vi "Log File.vi"(8 "Error In":errorcluster, 10 "Model (F-ME74)":bool, 11 "Test Data table":refnum<vi>) -> (0 "Error Out":errorcluster)   [LabVIEW 2018]
uses:
  <vilib>/Utility/file.llb/Write Delimited Spreadsheet (string).vi
panel:
  # "LOG File"
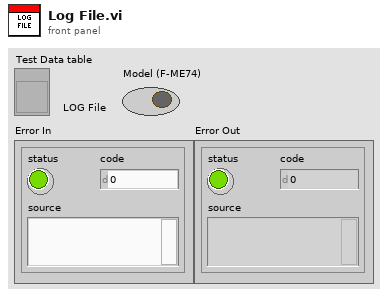
[diagram p1: front panel]
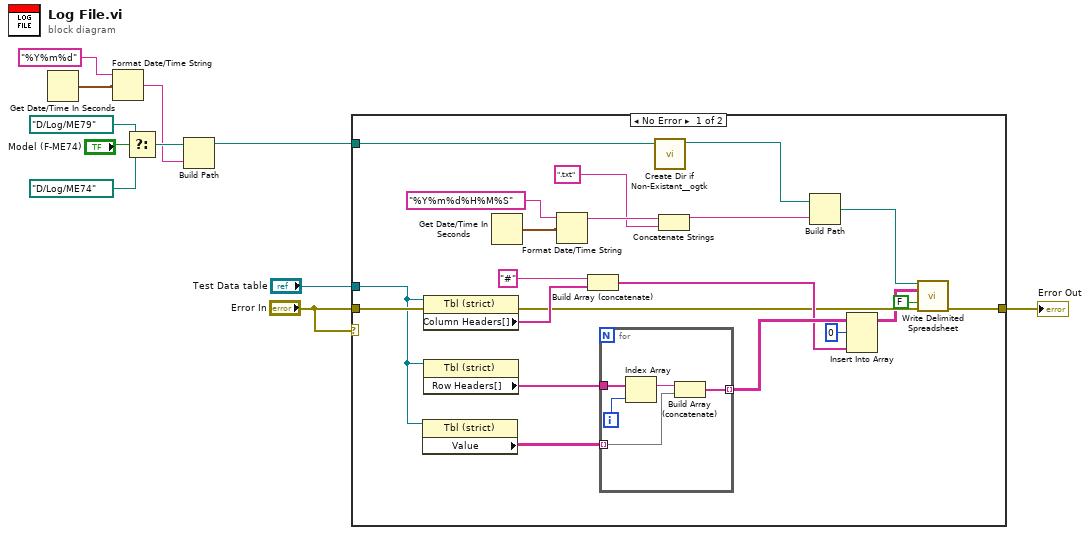
[diagram p0: block diagram]
diagram:
  n1 = Get Date/Time In Seconds() -> (seconds since 1Jan1904=w4:timestamp)
  n2 = Format Date/Time String(time format string (%c)="%Y%m%d", seconds (now)=w4) -> (date/time string=w2:string)  [unwired: 1 in]
  n3 = Select(t=path "D:/Log/ME79" ("base path"), s="Model (F-ME74)", f=path "D:/Log/ME74" ("base path")) -> (s? t:f=w3:path)
  n4 = Build Path(base path=w3, name or relative path=w2) -> (appended path=w1:path)
  n5 = case shown="No Error" "Error In" {
    tunnel: "Error In" -> [w32 w38]
    tunnel: "Test Data table" -> [w22 _]
    tunnel: [w21 w38] -> w10
    tunnel: w1 -> [w14 _]
    frame No Error {
      n6 = property class="Tbl (strict)"(reference=w22) -> ("Value"=w28:string[][])  [unwired: 1 in, 2 out]
      n7 = property class="Tbl (strict)"(reference=w22, error in=w32) -> (error out=w24:errorcluster, "Column Headers[]"=w30:string[])  [unwired: 1 out]
      n8 = property class="Tbl (strict)"(reference=w22) -> ("Row Headers[]"=w29:string[])  [unwired: 1 in, 2 out]
      n9 = Get Date/Time In Seconds() -> (seconds since 1Jan1904=w20:timestamp)
      n10 = Format Date/Time String(time format string (%c)="%Y%m%d%H%M%S", seconds (now)=w20) -> (date/time string=w18:string)  [unwired: 1 in]
      n11 = Build Array (concatenate)("#", w30) -> (w26:string[])
      n12 = for {
        tunnel: w28 -> [w33] mode=indexing
        tunnel: [w37] -> w27 mode=indexing
        tunnel: w29 -> [w36]
        i -> [w35]
        n13 = Index Array(array=w36, index=w35) -> (element=w34:string)
        n14 = Build Array (concatenate)(w34, w33) -> (w37:string[])
      }
      n15 = call <userlib>:"Create Dir if Non-Existant__ogtk.vi"("Directory Path"=w14) -> ("dup Directory Path"=w13:path)  [unwired: 8 in, 2 out]
      n16 = Concatenate Strings(w18, ".txt") -> (w16:string)
      n17 = Build Path(base path=w13, name or relative path=w16) -> (appended path=w12:path)
      n18 = Insert Into Array(array=w27, index (row)=0, new element=w26) -> (w23:string[][])  [unwired: 1 in]
      n19 = call-poly <vilib>:"Write Delimited Spreadsheet.vi"("file path (dialog if empty)"=w12, "2D data"=w23, "append to file? (new file:F)"=FALSE, "error in (no error)"=w24) -> ("error out"=w21:errorcluster)  [unwired: 10 in, 1 out]
    }
    frame Error {
    }
  }
  "Error Out" <- w10
